vi "Generate Signal From 1D Fourier Coefficients.vi"(10 "Samples":i32, 11 "Coefficients in":cluster{"A0":dbl, "Am":dbl[], "Bm":dbl[]}) -> (3 "Signal":dbl[](array[numeric]))   [LabVIEW 2020]
uses:
  <vilib>/Analysis/NI_AALBase.lvlib
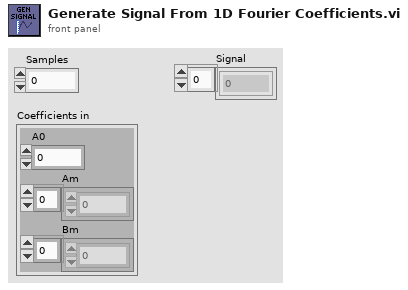
[diagram p1: front panel]
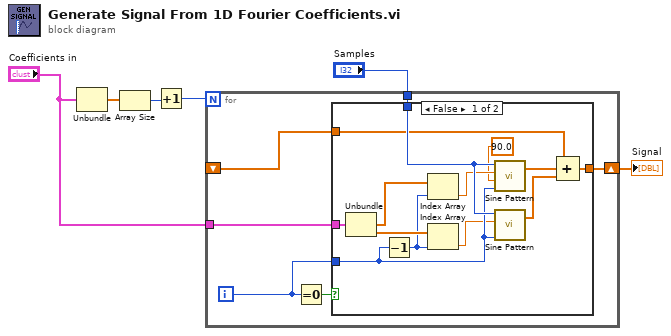
[diagram p0: block diagram]
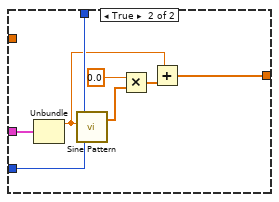
[diagram p2: hidden frame]
diagram:
  n1 = Unbundle("Coefficients in") -> ("Am"=w3:dbl[])  [unwired: 2 out]
  n2 = Array Size(array=w3) -> (size(s)=w2:i32)
  n3 = Increment(x=w2) -> (x+1=w1:i32)
  n4 = for {
    N: w1 -> [_]
    tunnel: "Samples" -> [w11]
    shift-right: [w10] -> w6
    shift-left: _ -> [w8]
    tunnel: "Coefficients in" -> [w9]
    i -> [w7]
    n5 = Equal To 0?(x=w7) -> (x = 0?=w12:bool)
    n6 = case shown="False" w12 {
      tunnel: w7 -> [w21 w33]
      tunnel: w11 -> [w25 w32]
      tunnel: [w13 w26] -> w10
      tunnel: w9 -> [w24 w31]
      tunnel: w8 -> [w14 _]
      frame False {
        n7 = Unbundle(w24) -> ("Am"=w23:dbl[], "Bm"=w22:dbl[])  [unwired: 1 out]
        n8 = Decrement(x=w21) -> (x-1=w20:i32)
        n9 = Index Array(array=w23, index=w20) -> (element=w19:dbl)
        n10 = Index Array(array=w22, index=w20) -> (element=w18:dbl)
        n11 = call <vilib>:"Sine Pattern.vi"("cycles"=w21, "phase(degrees)"=90.0, "amplitude"=w19, "samples"=w25) -> ("Sinusoidal Pattern"=w16:dbl[])  [unwired: 1 out]
        n12 = call <vilib>:"Sine Pattern.vi"("cycles"=w21, "amplitude"=w18, "samples"=w25) -> ("Sinusoidal Pattern"=w15:dbl[])  [unwired: 1 in, 1 out]
        n13 = Compound Arithmetic op=ADD(w14, w16, w15) -> (w13:dbl[])
      }
      frame True {
        n14 = Unbundle(w31) -> ("A0"=w27:dbl)  [unwired: 2 out]
        n15 = call <vilib>:"Sine Pattern.vi"("cycles"=w33, "amplitude"=w27, "samples"=w32) -> ("Sinusoidal Pattern"=w30:dbl[])  [unwired: 1 in, 1 out]
        n16 = Multiply(x=0.0, y=w30) -> (x*y=w28:dbl[])
        n17 = Add(x=w27, y=w28) -> (x+y=w26:dbl[])
      }
    }
  }
  "Signal" <- w6
